vi "set_motion_by_name.vi"(8 "error in (no error)":errorcluster caption="错误输入（无错误）", 9 "簇":T1, 10 "name":string, 11 "MotorSystem输入":refnum<class "MotorSystem.lvclass">) -> (0 "error out":errorcluster caption="错误输出", 3 "MotorSystem输出":refnum<class "MotorSystem.lvclass">)   [LabVIEW 2016, in "MotionControl_UFO_3DOF.lvlib" / "MotorSystem.lvclass"]
uses:
  <userlib>/MotionControl_UFO_3DOF/MotorSystem/MotorSystem.lvclass
  <userlib>/MotionControl_UFO_3DOF/MotorSystem/MotionCluster.ctl
  <userlib>/MotionControl_UFO_3DOF/OneMotion/OneMotion.lvclass
  <userlib>/MotionControl_UFO_3DOF/MotorSystem/MotorSystem.lvclass/MotorSystem.ctl
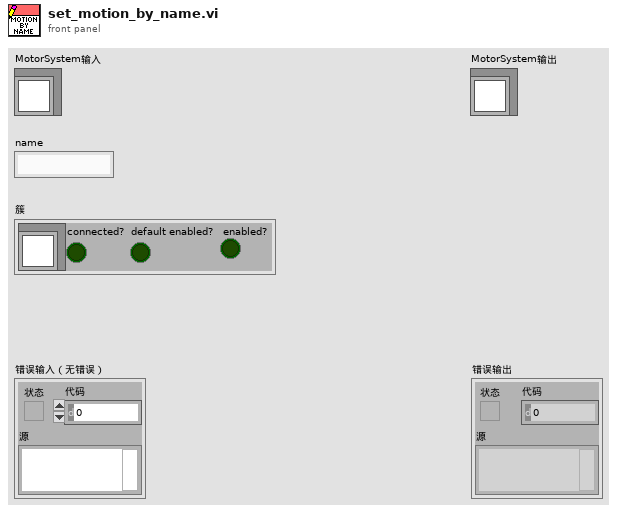
[diagram p1: front panel]
types:
  T1 = typedef "MotionControl_UFO_3DOF.lvlib/MotorSystem.lvclass/MotionCluster.ctl" = cluster{"OneMotion.lvclass":refnum<class "OneMotion.lvclass">, "connected?":bool, "default enabled?":bool, "enabled?":bool}
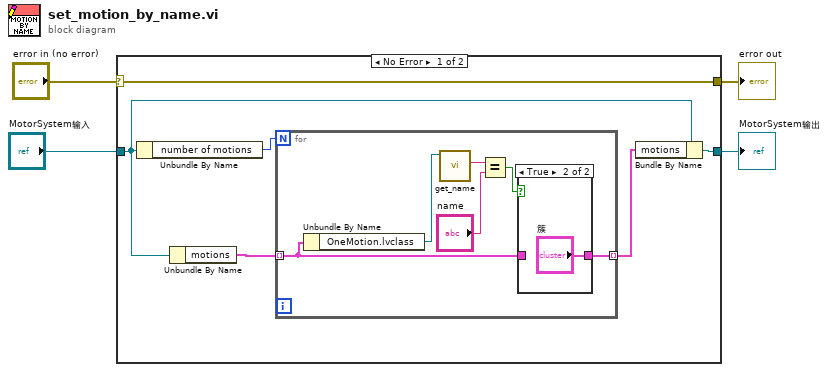
[diagram p0: block diagram]
diagram:
  n1 = case shown="No Error" "error in (no error)" {
    selector: "error in (no error)" -> [w10 w19]
    tunnel: [w10 w19] -> w3
    tunnel: [w9 w20] -> w1
    tunnel: "MotorSystem输入" -> [w8 w20]
    frame No Error {
      n2 = Unbundle By Name(w8) -> ("number of motions"=w7:i32)
      n3 = Unbundle By Name(w8) -> ("motions"=w6:T1[])
      n4 = for {
        N: w7 -> [_]
        tunnel: w6 -> [w12] mode=indexing
        tunnel: [w11] -> w5 mode=indexing
        n5 = Unbundle By Name(w12) -> ("OneMotion.lvclass"=w16:refnum<class "OneMotion.lvclass">)
        n6 = call-dynamic "get_name.vi"("OneMotion输入"=w16) -> ("name"=w15:string)  [unwired: 8 in, 2 out]
        n7 = Equal?(x=w15, y="name") -> (x = y?=w13:bool)
        n8 = case shown="True" w13 {
          tunnel: w12 -> [w17 _]
          tunnel: [w17 "簇"] -> w11
          frame False {
          }
          frame True {
          }
        }
      }
      n9 = Bundle By Name(cluster=w8, "motions"=w5) -> (w9:refnum<class "MotorSystem.lvclass">)
    }
    frame Error {
    }
  }
  "error out" <- w3
  "MotorSystem输出" <- w1
